vi "P1.vi"() -> ()   [LabVIEW 2013]
uses:
  <vilib>/measure/macond.llb/Continuous Waveform Convolution for 1 Chan.vi
  <vilib>/measure/NI_MABase.lvlib
  <vilib>/measure/NI_MAPro.lvlib
panel:
  out "Waveform Graph":waveform(dbl)(graph)
  in  "FRECUENCIA":dbl
  in  "NIVEL DE RUIDO":dbl
  in  "N":dbl
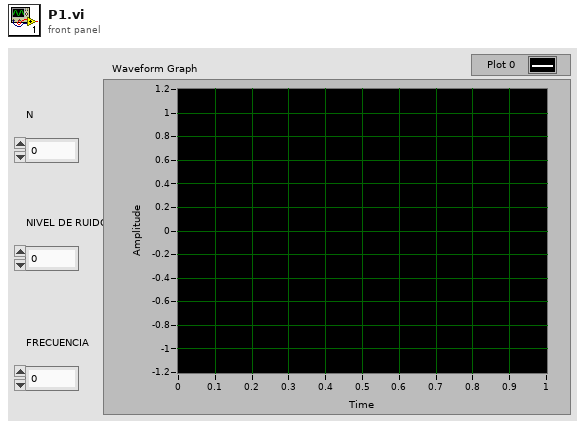
[diagram p1: front panel]
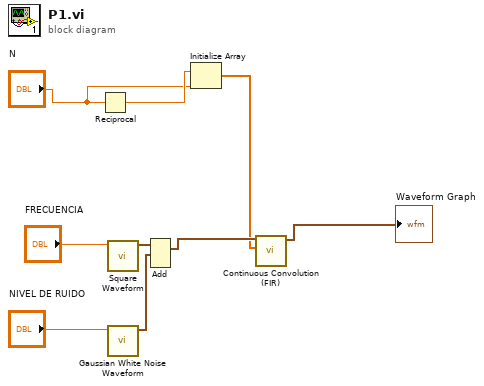
[diagram p0: block diagram]
diagram:
  n1 = Reciprocal(x="N") -> (1/x=w2:dbl)
  n2 = call <vilib>:"Square Waveform.vi"("frequency"="FRECUENCIA") -> ("signal out"=w7:waveform(dbl))  [unwired: 9 in, 1 out]
  n3 = call <vilib>:"Gaussian White Noise Waveform.vi"("standard deviation"="NIVEL DE RUIDO") -> ("signal out"=w6:waveform(dbl))  [unwired: 9 in, 1 out]
  n4 = Add(1:w6, 2:w7) -> (0:w5:waveform(dbl))  [unwired: 1 in, 1 out]
  n5 = Initialize Array(w2, "N") -> (w3:dbl[])
  n6 = call-poly <vilib>:"Continuous Convolution (FIR).vi"("kernel"=w3, "signal in"=w5) -> ("signal out"=→"Waveform Graph":waveform(dbl))  [unwired: 8 in, 1 out]
